vi "Global 5.vi"() -> ()   [LabVIEW 2015]
panel:
  in  "Read Buffer":string
  in  "Delay_eclipse":dbl
  in  "Eclipse_Load_Current":dbl
  in  "Load_Current_Step":dbl
  in  "i":dbl
  in  "Saved_Hour":dbl
  in  "IsEclipse":bool
  out "Channel2_OFF":bool
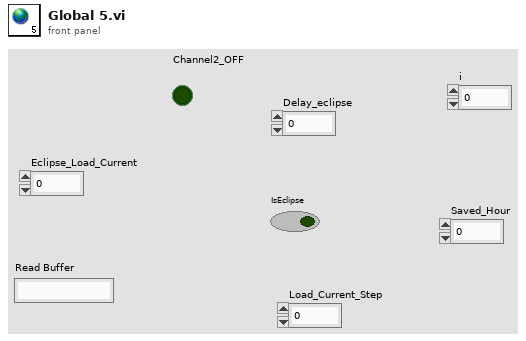
[diagram p1: front panel]
diagram:
